vi "check_command_type.vi"(11 "Current command":string) -> (0 "Wait for: __ milliseconds":u32, 3 "stop type":T1=enum."G4 all execution pause")   [LabVIEW 2017, in "labview-standard-library.lvlib" / "automode-scripting.lvlib"]
uses:
  automode-scripting.lvlib
  <vilib>/Utility/error.llb/whitespace.ctl
  type-defs/execution_stop_type.ctl
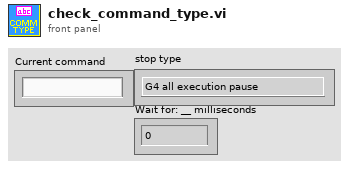
[diagram p1: front panel]
types:
  T1 = typedef "labview-standard-library.lvlib/automode-scripting.lvlib/execution_stop_type.ctl" = enum16{"G4 timed pause", "G4 all execution pause", "G4 single execution pause", "M0 Breakpoint", "Invalid"}
  T2 = typedef "whitespace.ctl" = u16
  T3 = typedef "execution_stop_type.ctl" = enum16{"G4 timed pause", "G4 execution pause", "M0 Breakpoint", "None"}
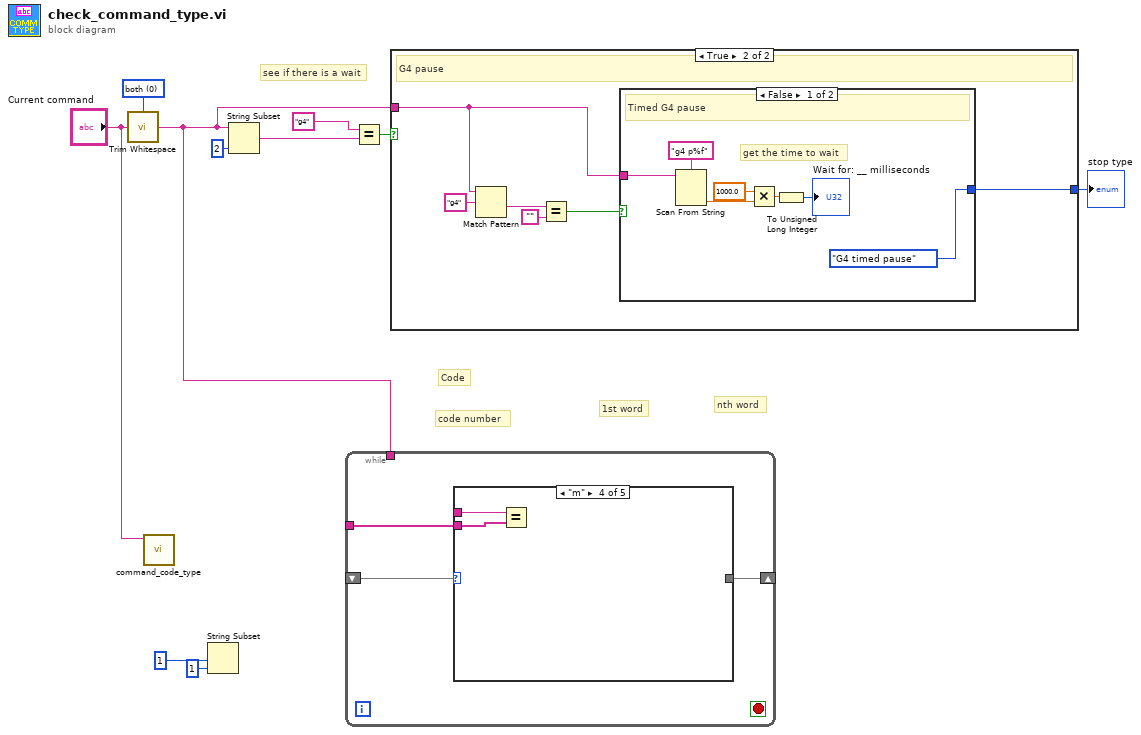
[diagram p0: block diagram]
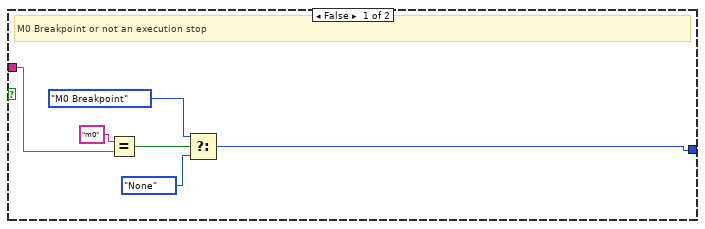
[diagram p6: hidden frame]
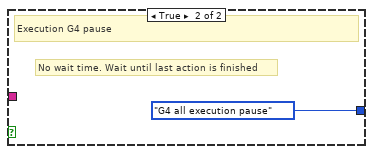
[diagram p7: hidden frame]
diagram:
  w9 = T2 0 items=["both", "start of string", "end of string"] ("location (both)")
  # "code number"
  # "nth word"
  # "1st word"
  # "Code"
  # "see if there is a wait"
  n1 = call <vilib>:"Trim Whitespace.vi"("string"="Current command", "location (both)"=w9) -> ("trimmed string"=w4:string)
  n2 = call "command_code_type.vi"("Line in"="Current command") -> ()  [unwired: 9 in, 2 out]
  n3 = String Subset(offset (0)=1, length (rest)=1 ("length (rest)")) -> ()  [unwired: 1 in, 1 out]
  n4 = String Subset(string=w4, length (rest)=2 ("length (rest)")) -> (substring=w5:string)  [unwired: 1 in]
  n5 = while {
    tunnel: _ -> [w11]
    shift-right: [w12] -> _
    shift-left: _ -> [w13]
    tunnel: w4 -> [_]
    stop <- _ stop-if-true
    n6 = case shown="\"m\"" w13 {
      tunnel: [_ _ _ _ _] -> w12
      tunnel: _ -> [_ _ _ w14 _]
      tunnel: w11 -> [_ _ _ w15 _]
      frame "init", Default {
      }
      frame "invalid" {
      }
      frame "g" {
      }
      frame "m" {
        n7 = Equal?(x=w14, y=w15) -> ()  [unwired: 1 out]
      }
      frame "t" {
      }
    }
  }
  n8 = Equal?(x="g4", y=w5) -> (x = y?=w7:bool)
  n9 = case shown="True" w7 {
    tunnel: [w17 w23] -> w6
    tunnel: w4 -> [w16 w22]
    frame False {
      # "M0 Breakpoint or not an execution stop"
      n10 = Equal?(x="m0", y=w16) -> (x = y?=w20:bool)
      n11 = Select(t=execution_stop_type."M0 Breakpoint", s=w20, f=execution_stop_type."None") -> (s? t:f=w17:u16)
    }
    frame True {
      # "G4 pause"
      n12 = Match Pattern(string=w22, regular expression="g4") -> (after substring=w26:string)  [unwired: 1 in, 3 out]
      n13 = Equal?(x=w26, y="") -> (x = y?=w24:bool)
      n14 = case shown="False" w24 {
        tunnel: w22 -> [w33 _]
        tunnel: [execution_stop_type."G4 timed pause" execution_stop_type."G4 all execution pause"] -> w23
        frame False {
          # "get the time to wait"
          # "Timed G4 pause"
          n15 = Scan From String(format string="g4 p%f", input string=w33) -> (output 1=w31:dbl)  [unwired: 3 in, 3 out]
          n16 = Multiply(x=1000.0, y=w31) -> (x*y=w29:dbl)
          n17 = To Unsigned Long Integer(number=w29) -> (unsigned 32bit integer=→"Wait for: __ milliseconds":u32)
        }
        frame True {
          # "No wait time. Wait until last action is finished"
          # "Execution G4 pause"
        }
      }
    }
  }
  "stop type" <- w6
